vi "Set Power Regulation.vi"(0 "shared in":refnum<class "niUSRP Rx Core v1 FPGA.lvclass">=refnum, 5 "power regulation":refnum<class "niVST Power Regulation v1 FPGA.lvclass">=refnum) -> (4 "shared out":refnum<class "niUSRP Rx Core v1 FPGA.lvclass">)   [LabVIEW 2023]
uses:
  <instrlib>/niVST/Power Regulation/Interface/v1/FPGA/niVST Power Regulation v1 FPGA.lvclass
  <instrlib>/niUSRP/Reference FPGA/Rx Core/niUSRP Rx Core v1 FPGA.lvclass
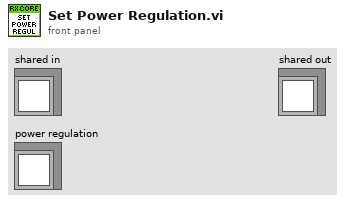
[diagram p1: front panel]
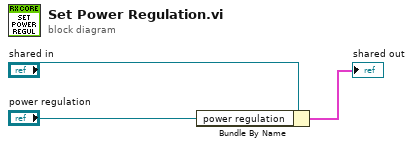
[diagram p0: block diagram]
diagram:
  n1 = Bundle By Name(cluster="shared in", "power regulation"="power regulation") -> (→"shared out":cluster{})
